vi "testAppendErrorInformation_NoError_withState.vi"(8 "error in (no error)":errorcluster, 11 "testStateMachineUtilities in":refnum<class "testStateMachineUtilities.lvclass">) -> (0 "error out":errorcluster, 3 "testStateMachineUtilities out":refnum<class "testStateMachineUtilities.lvclass">)   [LabVIEW 2020, in "testStateMachineUtilities.lvclass"]
uses:
  testStateMachineUtilities.lvclass
  source/State Machine Support API/Parse State Queue_2024.vi
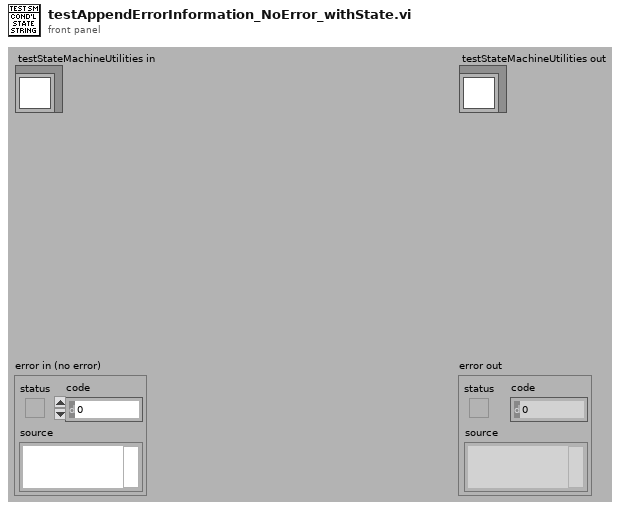
[diagram p1: front panel]
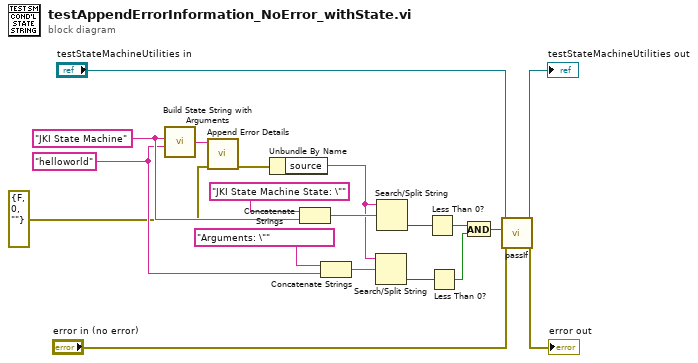
[diagram p0: block diagram]
diagram:
  w17 = "JKI State Machine" ("Previous State and Argument(s)")
  w11 = "helloworld" ("Previous State and Argument(s)")
  n1 = call "Build State String with Arguments.vi"("Arguments (\"\")"=w11, "State"=w17) -> ("State with Arguments"=w19:string)  [unwired: 4 in]
  n2 = call "Append Error Details.vi"("error in (no error)"=errorcluster {"status"=FALSE, "code"=0, "source"=""}, "Previous State and Argument(s)"=w19) -> ("error out"=w3:errorcluster)  [unwired: 9 in]
  n3 = Unbundle By Name(w3) -> ("source"=w2:string)
  n4 = Concatenate Strings("JKI State Machine State: \"" ("search string/char (-)"), w17) -> (w8:string)
  n5 = Concatenate Strings("Arguments: \"" ("search string/char (-)"), w11) -> (w7:string)
  n6 = Search/Split String(string=w2, search string/char (-)=w7) -> (offset of match=w9:i32)  [unwired: 1 in, 2 out]
  n7 = Search/Split String(string=w2, search string/char (-)=w8) -> (offset of match=w12:i32)  [unwired: 1 in, 2 out]
  n8 = Less Than 0?(x=w12) -> (x < 0?=w6:bool)
  n9 = Less Than 0?(x=w9) -> (x < 0?=w5:bool)
  n10 = And(x=w6, y=w5) -> (x .and. y?=w4:bool)
  n11 = call-dynamic "passIf.vi"("error in (no error)"="error in (no error)", "pass"=w4, "TestCase in"="testStateMachineUtilities in") -> ("error out"=→"error out":errorcluster, "TestCase out"=→"testStateMachineUtilities out":refnum<class "testStateMachineUtilities.lvclass">)  [unwired: 7 in]
